vi "Convert_to_2009.vi"(8 "error in (no error)":errorcluster, 11 "userFolder in":refnum<class "userFolder.lvclass">) -> (0 "error out":errorcluster, 2 "preserve?":bool, 3 "DirInfo":T1)   [LabVIEW 2020, in "userFolder.lvclass"]
uses:
  <vilib>/AppBuilder/IB_Classes/Destination/userFolder/userFolder.lvclass
  <vilib>/AppBuilder/IB_Classes/Destination/userFolder/userFolder.lvclass/userFolder.ctl
  <resource>/Framework/Providers/Builds/Installer/CDK_sTypeDef_DirInfo.ctl
  <vilib>/AppBuilder/IB_Classes/Destination/IB_Destination.lvclass
  e:/builds/penguin/labview/branches/2020/dev/dist/vi.lib/AppBuilder/IB_Classes/Destination/IB_Destination.lvclass
  e:/builds/penguin/labview/branches/2020/dev/dist/vi.lib/AppBuilder/IB_Classes/Destination/userFolder/userFolder.lvclass
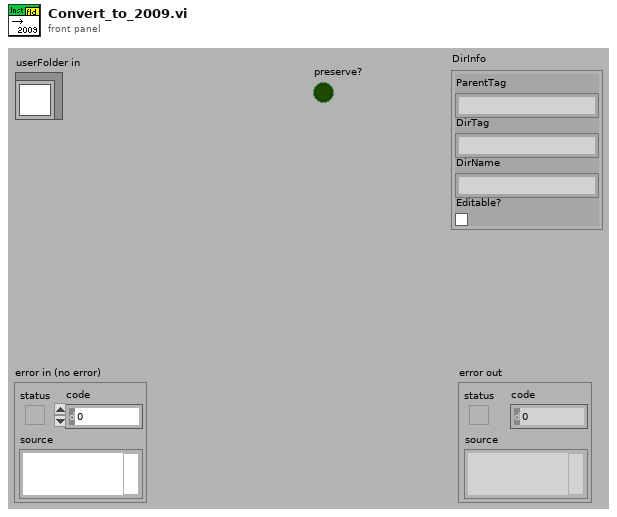
[diagram p1: front panel]
types:
  T1 = typedef "CDK_sTypeDef_DirInfo.ctl" = cluster{"ParentTag":string, "DirTag":string, "DirName":string, "Editable?":bool}
  T2 = typedef "IB_Destination.ctl" = cluster{"name":string, "unlock":bool, "parentTag":string, "destTag":string, "eng_installPath":string}
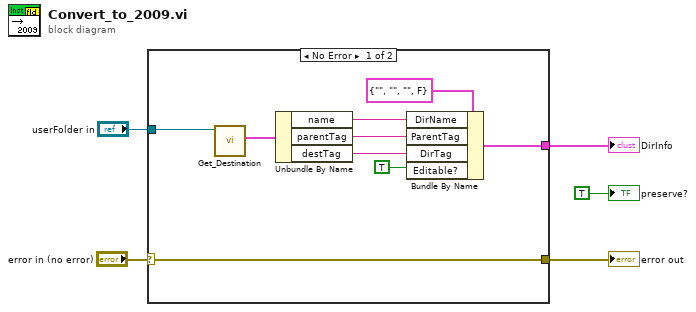
[diagram p0: block diagram]
diagram:
  n1 = case shown="No Error" "error in (no error)" {
    selector: "error in (no error)" -> [w6 w15]
    tunnel: "userFolder in" -> [w9 _]
    tunnel: [w7 _] -> w4
    tunnel: [w6 w15] -> w1
    frame No Error {
      n2 = call <vilib>:"Get_Destination.vi"("IB_Destination in"=w9) -> ("data"=w8:T2)  [unwired: 1 in, 9 out]
      n3 = Unbundle By Name(w8) -> ("name"=w10:string, "parentTag"=w11:string, "destTag"=w12:string)
      n4 = Bundle By Name(cluster=T1 {"ParentTag"="", "DirTag"="", "DirName"="", "Editable?"=FALSE} ("DirInfo"), "DirName"=w10, "ParentTag"=w11, "DirTag"=w12, "Editable?"=TRUE) -> (w7:T1)
    }
    frame Error {
    }
  }
  "error out" <- w1
  "DirInfo" <- w4
  "preserve?" <- TRUE ("preserve?")
